vi "5 collaudi.vi"(11 "CURVE SINGOLE in":T1) -> (3 "Curve singole out":T1)   [LabVIEW 2016]
uses:
  TypeDef/Curve singole.ctl
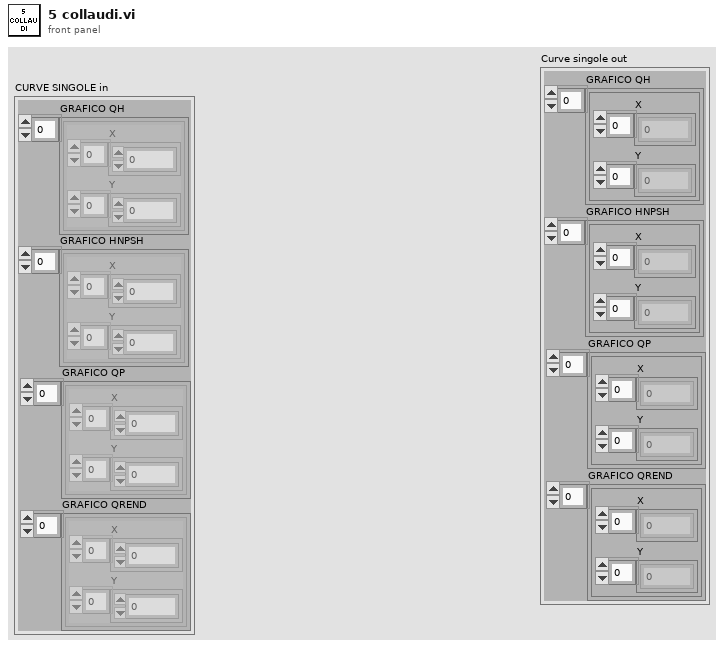
[diagram p1: front panel]
types:
  T1 = typedef "Curve singole.ctl" = cluster{"GRAFICO QH":cluster{"X":dbl[], "Y":dbl[]}[], "GRAFICO HNPSH":cluster{"X":dbl[], "Y":dbl[]}[], "GRAFICO QP":cluster{"X":dbl[], "Y":dbl[]}[], "GRAFICO QREND":cluster{"X":dbl[], "Y":dbl[]}[]}
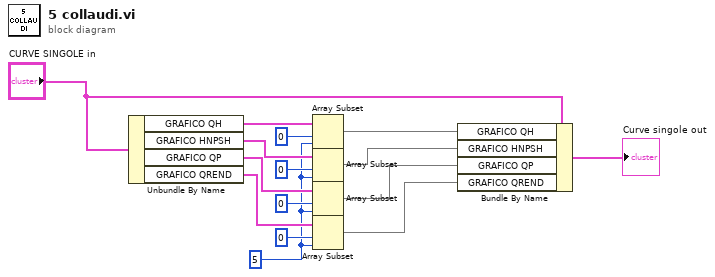
[diagram p0: block diagram]
diagram:
  w7 = 5 ("index")
  n1 = Unbundle By Name("CURVE SINGOLE in") -> ("GRAFICO QH"=w15:cluster{"X":dbl[], "Y":dbl[]}[], "GRAFICO HNPSH"=w14:cluster{"X":dbl[], "Y":dbl[]}[], "GRAFICO QP"=w13:cluster{"X":dbl[], "Y":dbl[]}[], "GRAFICO QREND"=w12:cluster{"X":dbl[], "Y":dbl[]}[])
  n2 = Array Subset(array=w15, index=0, length=w7) -> (w5:cluster{"X":dbl[], "Y":dbl[]}[])
  n3 = Array Subset(array=w14, index=0, length=w7) -> (w4:cluster{"X":dbl[], "Y":dbl[]}[])
  n4 = Array Subset(array=w13, index=0, length=w7) -> (w3:cluster{"X":dbl[], "Y":dbl[]}[])
  n5 = Array Subset(array=w12, index=0, length=w7) -> (w2:cluster{"X":dbl[], "Y":dbl[]}[])
  n6 = Bundle By Name(cluster="CURVE SINGOLE in", "GRAFICO QH"=w5, "GRAFICO HNPSH"=w4, "GRAFICO QP"=w3, "GRAFICO QREND"=w2) -> (→"Curve singole out":T1)
